vi "get_beta.vi"(1 "Data Rate [Hz]":dbl, 2 "Time Constant [s]":dbl) -> (0 "beta":i32)   [LabVIEW 2009]
doc: "Gets beta (1 pole filter parameter). Inputs are time constant tau [s] and data rate R [Hz]."
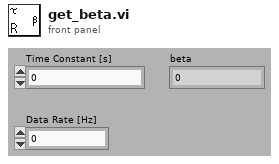
[diagram p1: front panel]
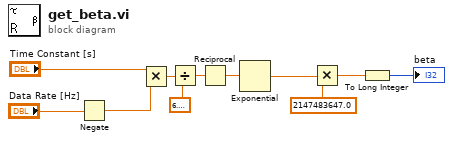
[diagram p0: block diagram]
diagram:
  n1 = Negate(x="Data Rate [Hz]") -> (-x=w6:dbl)
  n2 = Multiply(x="Time Constant [s]", y=w6) -> (x*y=w3:dbl)
  n3 = Divide(x=w3, y=6.283185307179586) -> (x/y=w2:dbl)
  n4 = Reciprocal(x=w2) -> (1/x=w8:dbl)
  n5 = Exponential(1:w8) -> (0:w10:dbl)
  n6 = Multiply(x=w10, y=2147483647.0) -> (x*y=w9:dbl)
  n7 = To Long Integer(number=w9) -> (32bit integer=→"beta":i32)
